vi "KeyPress.vi"(0 "Virtual Key":u8(ring)=65, 7 "Millis":u32, 11 "error in":errorcluster) -> (15 "error out":errorcluster)   [LabVIEW 2016, in "Drona.lvlib" / "KeyboardSimulation.lvlib"]
doc: "Press the key down then up"
uses:
  KeyboardSimulation.lvlib
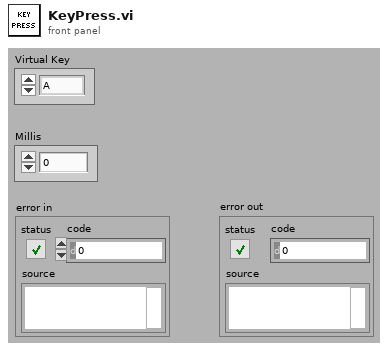
[diagram p1: front panel]
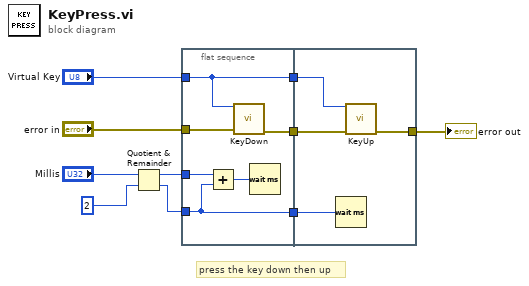
[diagram p0: block diagram]
diagram:
  # "press the key down then up"
  n1 = Quotient & Remainder(x="Millis", y=u32 2) -> (x-y*floor(x/y)=w6:u32, floor(x/y)=w5:u32)
  n2 = flat-sequence {
    tunnel: "Virtual Key" -> [w14]
    tunnel: [w14] -> w9
    tunnel: w6 -> [w16]
    tunnel: w5 -> [w13]
    tunnel: [w13] -> w4
    tunnel: [w12] -> w3
    tunnel: "error in" -> [w11]
    tunnel: w9 -> [w20]
    tunnel: w4 -> [w19]
    tunnel: w3 -> [w18]
    tunnel: [w17] -> w1
    frame #0 {
      n3 = Add(x=w16, y=w13) -> (x+y=w15:u32)
      n4 = call "KeyDown.vi"("Virtual Key"=w14, "error in"=w11) -> ("error out"=w12:errorcluster)  [unwired: 13 in]
      n5 = Wait (ms)(milliseconds to wait=w15) -> ()  [unwired: 1 out]
    }
    frame #1 {
      n6 = Wait (ms)(milliseconds to wait=w19) -> ()  [unwired: 1 out]
      n7 = call "KeyUp.vi"("Virtual Key"=w20, "error in"=w18) -> ("error out"=w17:errorcluster)  [unwired: 13 in]
    }
  }
  "error out" <- w1
